vi "OFET2.vi"() -> ()   [LabVIEW 2017]
uses:
  EnumEstados1.ctl
  <vilib>/Analysis/3filter.llb/Filter Passband Type.ctl
  <vilib>/Analysis/baseanly.llb/IIR Cascade Filter (DBL).vi
  <vilib>/Analysis/NI_AALBase.lvlib
  <vilib>/Utility/NIReport.llb/NI_report.lvclass
  <vilib>/addons/_office/NI_ReportGenerationToolkit.lvlib
  <vilib>/addons/_office/excel.llb/Excel Easy Table (str).vi
panel:
  in  "Tab Control":T1(tab)
  in  "Voltaje final:  2":dbl=5.0
  in  "Voltaje inicial:  2":dbl
  in  "Paso: 2":dbl
  in  "Voltaje final:":dbl=5.0
  in  "Voltaje inicial:":dbl
  in  "Paso:":dbl=0.1
  in  "Paso":dbl
  in  "Voltaje inicial:":dbl
  in  "Voltaje final:":dbl
  in  "Voltaje:":dbl
  in  "order":i32
  in  "Stop Button":bool
  in  "Save Button":bool
  in  "Guardar en:":path
  out "Voltage-Current Characterization:":cluster{dbl[], "Filtered X":dbl[]}(graph)
  in  "Ok":bool
  # "OFET"
  # "VGS"
  # "VDS"
  # "VGS"
  # "VDS"
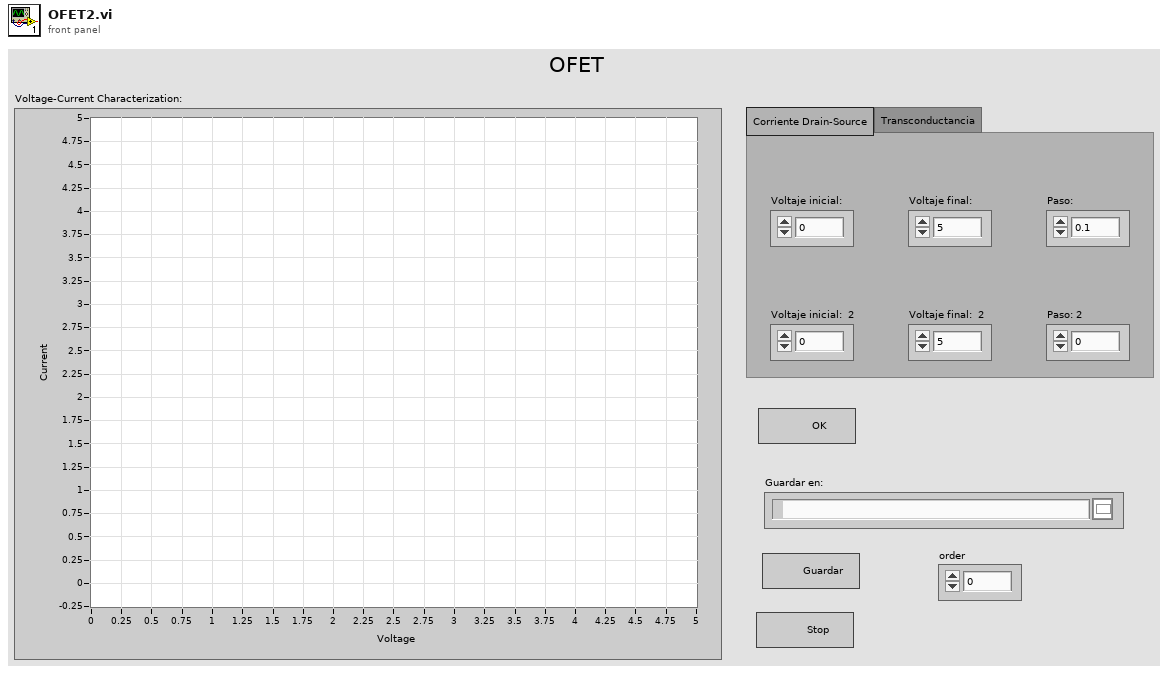
[diagram p1: front panel]
types:
  T1 = enum32{"Corriente Drain-Source", "Transconductancia"}
  T2 = typedef "EnumEstados1.ctl" = enum16{"Inicio", "LecturaDatos", "Cierre"}
  T3 = typedef "NI_AALBase.lvlib/Filter Passband Type.ctl" = enum32{"Lowpass", "Highpass", "Bandpass", "Bandstop"}
  T4 = enum16{"Standard Report", "HTML", "Word", "Excel"}
  T5 = enum16{"maximized", "minimized", "normal", "no change"}
  T6 = enum16{"open", "open or create", "create or replace", "create", "open (read-only)"}
  T7 = cluster{"task out":refnum<k21>, "error out":errorcluster}
  T8 = cluster{"filter structure":enum32{"IIR 2nd Order", "IIR 4th Order"}, "Reverse Coefficients":dbl[], "Forward Coefficients":dbl[]}
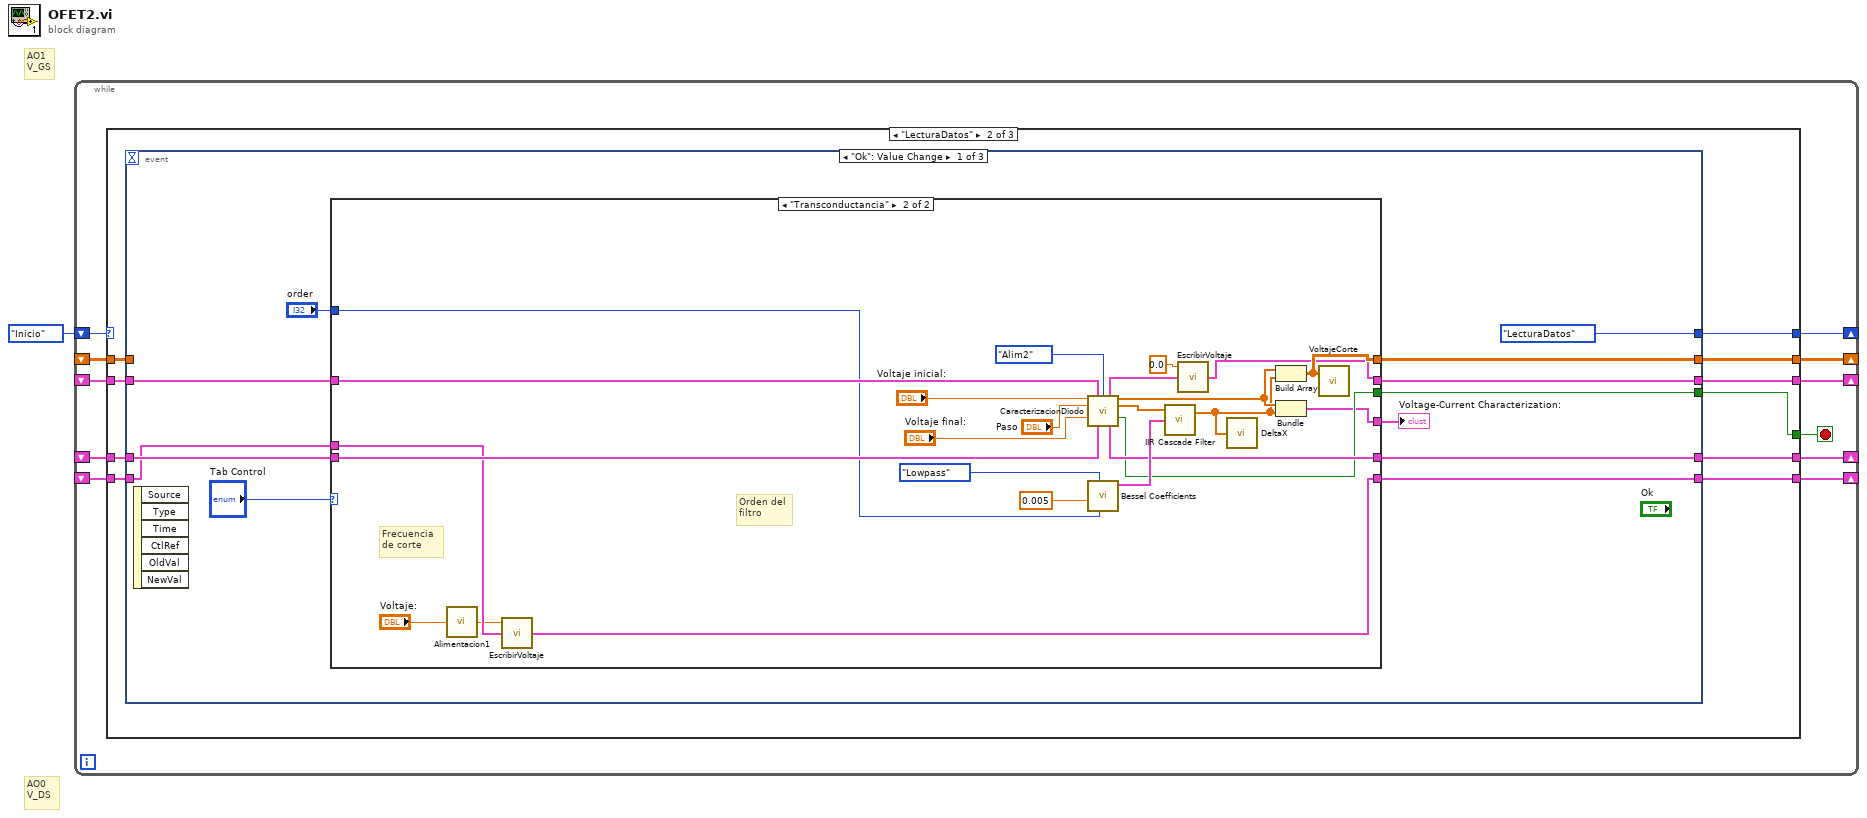
[diagram p0: block diagram]
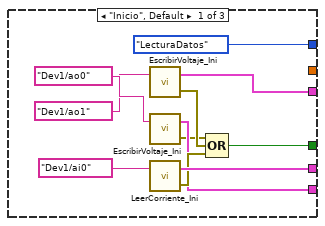
[diagram p2: hidden frame]
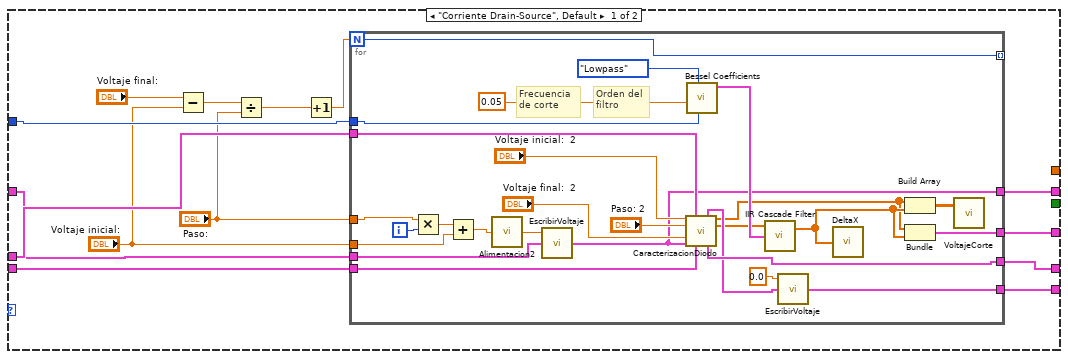
[diagram p3: hidden frame]
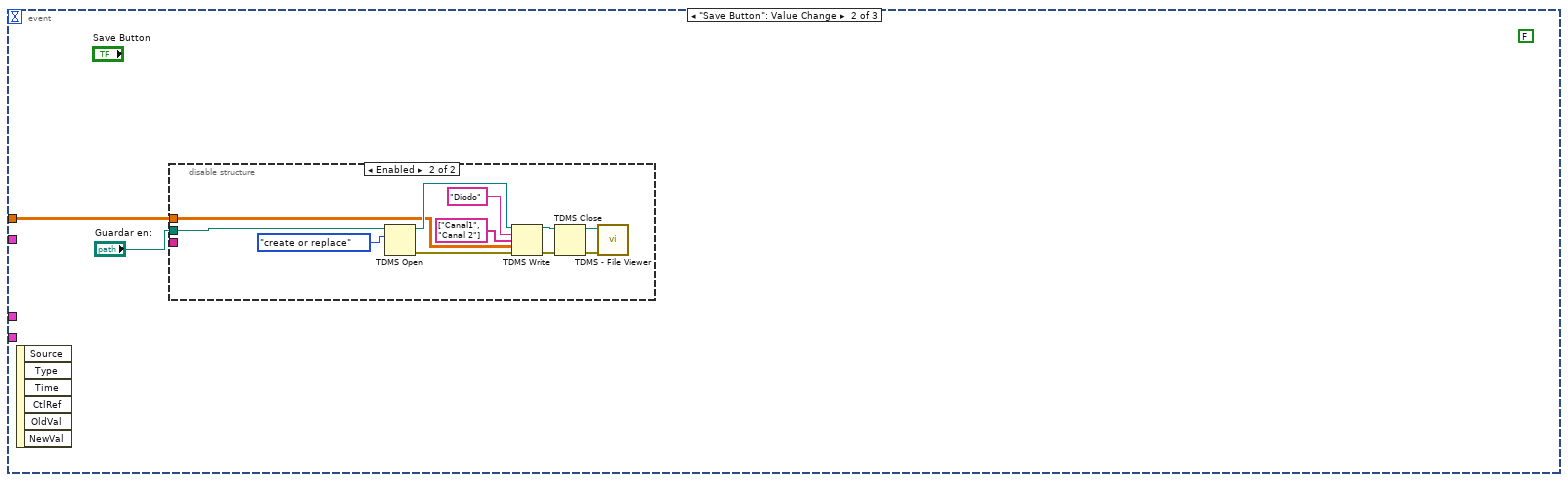
[diagram p4: hidden frame]
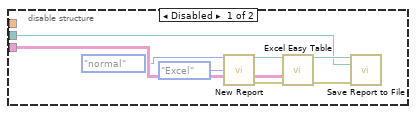
[diagram p5: hidden frame]
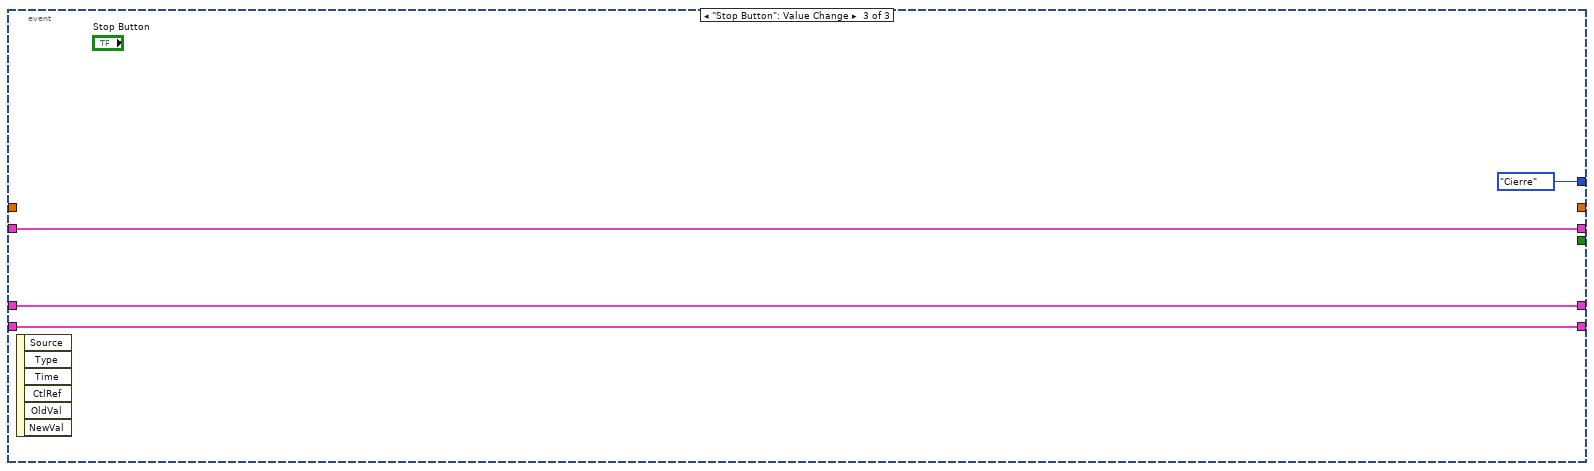
[diagram p6: hidden frame]
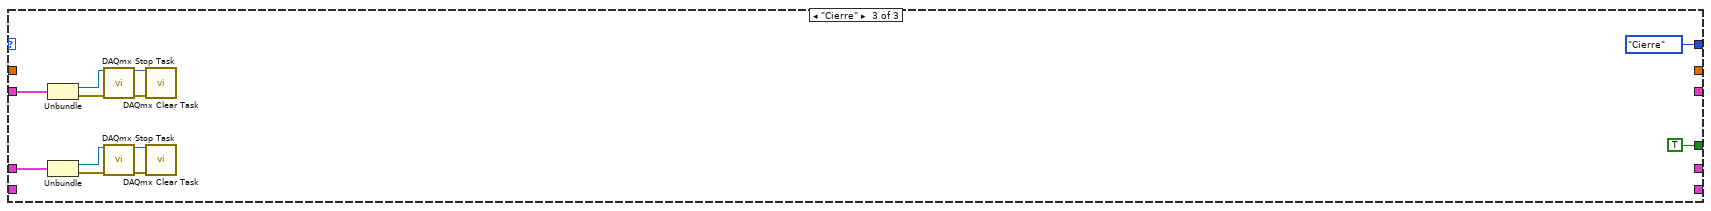
[diagram p7: hidden frame]
diagram:
  # "AO1\nV_GS"
  # "AO0\nV_DS"
  n1 = while {
    shift-right: [w7] -> _
    shift-left: EnumEstados1."Inicio" -> [w12]
    shift-right: [w11] -> _
    shift-left: _ -> [w10]
    shift-right: [w9] -> _
    shift-left: _ -> [w8]
    shift-right: [w6] -> _
    shift-left: _ -> [w5]
    shift-right: [w3] -> _
    shift-left: _ -> [w2]
    stop <- w4 stop-if-true
    n2 = case shown="\"LecturaDatos\"" w12 {
      tunnel: [w22 w32 _] -> w11
      tunnel: w10 -> [_ w33 w143]
      tunnel: [w21 w30 _] -> w9
      tunnel: w8 -> [_ w31 w142]
      tunnel: [EnumEstados1."LecturaDatos" w29 EnumEstados1."Cierre"] -> w7
      tunnel: [_ w28 _] -> w6
      tunnel: w5 -> [_ w27 _]
      tunnel: [w18 w26 TRUE] -> w4
      tunnel: [w17 w24 _] -> w3
      tunnel: w2 -> [_ w25 _]
      frame "Inicio", Default {
        n3 = call "EscribirVoltaje_Ini.vi"("physical channels"=tag "Dev1/ao1") -> ("error out"=w20:errorcluster, "cluster"=w22:T7)  [unwired: 1 in]
        n4 = call "EscribirVoltaje_Ini.vi"("physical channels"=tag "Dev1/ao0") -> ("error out"=w16:errorcluster, "cluster"=w17:T7)  [unwired: 1 in]
        n5 = call "LeerCorriente_Ini.vi"("physical channels"=tag "Dev1/ai0") -> ("error out"=w19:errorcluster, "output cluster"=w21:T7)  [unwired: 1 in]
        n6 = Compound Arithmetic op=OR(w16, w20, w19) -> (w18:bool)
      }
      frame "LecturaDatos" {
        n7 = event shown="[0] \"Ok\": Value Change" {
          selector: _ -> [_ _ _]
          dyn-events: _ -> [_ _ _]
          timeout: _ -> [_ _ _]
          tunnel: w33 -> [w44 _ w135]
          tunnel: [w37 _ w135] -> w32
          tunnel: w31 -> [w43 _ w134]
          tunnel: [w42 _ w134] -> w30
          tunnel: [EnumEstados1."LecturaDatos" _ EnumEstados1."Cierre"] -> w29
          tunnel: [w40 _ _] -> w28
          tunnel: w27 -> [_ w111 _]
          tunnel: [w41 _ _] -> w26
          tunnel: w25 -> [w39 _ w132]
          tunnel: [w38 _ w132] -> w24
          event "Ok": Value Change {
            n8 = event-data() -> ()  [unwired: 1 in, 6 out]
            n9 = case shown="\"Transconductancia\"" "Tab Control" {
              tunnel: w44 -> [w53 w108]
              tunnel: w43 -> [w57 w107]
              tunnel: [w56 w106] -> w42
              tunnel: [_ w105] -> w41
              tunnel: [_ w104] -> w40
              tunnel: w39 -> [w58 w100]
              tunnel: [w55 w99] -> w38
              tunnel: [w52 w97] -> w37
              tunnel: "order" -> [w59 w91]
              tunnel: [w54 w90] -> w34
              frame "Corriente Drain-Source", Default {
                n10 = Subtract(x="Voltaje final:", y="Voltaje inicial:") -> (x-y=w50:dbl)
                n11 = Divide(x=w50, y="Paso:") -> (x/y=w49:dbl)
                n12 = Increment(x=w49) -> (x+1=w46:dbl)
                n13 = for {
                  N: w46 -> [w66]
                  tunnel: w59 -> [w81]
                  tunnel: w58 -> [w77]
                  tunnel: w57 -> [w76]
                  tunnel: [w75] -> w56
                  tunnel: [w73] -> w55
                  tunnel: [w69] -> w54
                  tunnel: w53 -> [w68]
                  tunnel: [w67] -> w52
                  tunnel: [w66] -> _ mode=indexing
                  tunnel: "Paso:" -> [w65]
                  tunnel: "Voltaje inicial:" -> [w62]
                  i -> [w64]
                  # "Frecuencia \nde corte"
                  # "Orden del\nfiltro"
                  n14 = Multiply(x=w65, y=w64) -> (x*y=w63:dbl)
                  n15 = Add(x=w63, y=w62) -> (x+y=w61:dbl)
                  n16 = call "Alimentacion2.vi"("VoltajeDeseado"=w61) -> ("Numeric Indicator"=w60:dbl)
                  n17 = call "EscribirVoltaje.vi"("cluster"=w68, "data"=w60) -> ("Cluster"=w67:T7)  [unwired: 1 in, 2 out]
                  n18 = call "CaracterizacionDiodo.vi"("Voltaje inicial:"="Voltaje inicial:  2", "Voltaje"=w77, "Paso"="Paso: 2", "Voltaje final:"="Voltaje final:  2", "Voltaje  2"=w67, "Corriente"=w76) -> (3:"Voltaje"=w74:T7, 4:"Voltaje"=w70:dbl[], 6:"Corriente"=w71:dbl[], 14:"Corriente"=w75:T7)  [unwired: 5 in, 1 out]
                  n19 = call <vilib>:"Bessel Coefficients.vi"("order"=w81, "filter type"=Filter_Passband_Type."Lowpass", "low cutoff freq: fl"=0.05 ("Numeric Control")) -> ("IIR Filter Cluster"=w86:T8)  [unwired: 7 in, 1 out]
                  n20 = call-poly <vilib>:"IIR Cascade Filter.vi"("IIR Filter Cluster"=w86, "X"=w71) -> ("Filtered X"=w83:dbl[])  [unwired: 1 in, 1 out]
                  n21 = call "EscribirVoltaje.vi"("cluster"=w74, "data"=0.0) -> ("Cluster"=w73:T7)  [unwired: 1 in, 2 out]
                  n22 = call "DeltaX.vi"("Array in"=w83) -> ()  [unwired: 1 out]
                  n23 = Build Array(w70, w83) -> (w84:dbl[][])
                  n24 = Bundle("Voltaje"=w70, "Filtered X"=w83) -> (w69:cluster{"Voltaje":dbl[], "Filtered X":dbl[]})  [unwired: 1 in]
                  n25 = call "VoltajeCorte.vi"("Array in"=w84) -> ()  [unwired: 1 in, 2 out]
                }
              }
              frame "Transconductancia" {
                # "Frecuencia \nde corte"
                # "Orden del\nfiltro"
                n26 = call "Alimentacion1.vi"("VoltajeDeseado"="Voltaje:") -> ("Numeric Indicator"=w88:dbl)
                n27 = call "EscribirVoltaje.vi"("cluster"=w100, "data"=w88) -> ("Cluster"=w99:T7)  [unwired: 1 in, 2 out]
                n28 = call "CaracterizacionDiodo.vi"("Voltaje inicial:"="Voltaje inicial:", "Voltaje"=w108, "Enum"=enum16{"Alim1", "Alim2"}."Alim2", "Paso"="Paso", "Voltaje final:"="Voltaje final:", "Corriente"=w107) -> (3:"Voltaje"=w98:T7, 4:"Voltaje"=w103:dbl[], 6:"Corriente"=w95:dbl[], "Error?"=w105:bool, 14:"Corriente"=w106:T7)  [unwired: 5 in]
                n29 = call <vilib>:"Bessel Coefficients.vi"("order"=w91, "filter type"=Filter_Passband_Type."Lowpass", "low cutoff freq: fl"=0.005 ("Numeric Control")) -> ("IIR Filter Cluster"=w110:T8)  [unwired: 7 in, 1 out]
                n30 = call-poly <vilib>:"IIR Cascade Filter.vi"("IIR Filter Cluster"=w110, "X"=w95) -> ("Filtered X"=w102:dbl[])  [unwired: 1 in, 1 out]
                n31 = call "EscribirVoltaje.vi"("cluster"=w98, "data"=0.0) -> ("Cluster"=w97:T7)  [unwired: 1 in, 2 out]
                n32 = call "DeltaX.vi"("Array in"=w102) -> ()  [unwired: 1 out]
                n33 = Build Array(w103, w102) -> (w104:dbl[][])
                n34 = Bundle("Voltaje"=w103, "Filtered X"=w102) -> (w90:cluster{"Voltaje":dbl[], "Filtered X":dbl[]})  [unwired: 1 in]
                n35 = call "VoltajeCorte.vi"("Array in"=w104) -> ()  [unwired: 1 in, 2 out]
              }
            }
            "Voltage-Current Characterization:" <- w34
          }
          event "Save Button": Value Change {
            (unwired) FALSE
            n36 = event-data() -> ()  [unwired: 1 in, 6 out]
            n37 = disable-structure shown="Enabled" {
              disable-tunnel: _ -> [w118 _]
              disable-tunnel: "Guardar en:" -> [w113 w124]
              disable-tunnel: w111 -> [_ w121]
              frame Disabled {
                n38 = call <vilib>:"New Report.vi"("window state (normal)"=T5."normal", "report type"=T4."Excel") -> ("report out"=w120:refnum<class "NI_report.lvclass">, "error out"=w119:errorcluster)  [unwired: 12 in]
                n39 = call-poly <vilib>:"Excel Easy Table.vi"("report in"=w120, "text data"=w118, "error in (no error)"=w119) -> ("report out"=w117:refnum<class "NI_report.lvclass">, "error out"=w116:errorcluster)  [unwired: 8 in, 3 out]
                n40 = call-dynamic "Save Report to File.vi"("report in"=w117, "report file path"=w113, "error in (no error)"=w116) -> ()  [unwired: 11 in, 2 out]
              }
              frame Enabled {
                n41 = TDMS Open(10:T6."create or replace" ("operation (0:open)"), 11:w124) -> (0:w128:errorcluster, 3:w125:refnum<k34>)  [unwired: 5 in]
                n42 = TDMS Write(0:w125, 5:"Diodo" ("group name in (Untitled)"), 7:string[] ["Canal1", "Canal 2"] ("channel name(s) in (Untitled)"), 9:w121, 11:w128) -> (4:w126:refnum<k34>, 15:w127:errorcluster)  [unwired: 1 in, 2 out]
                n43 = TDMS Close(8:w127, 11:w126) -> (0:w123:errorcluster, 3:w122:path)
                n44 = call <vilib>:"TDMS - File Viewer.vi"("error in (no error)"=w123, "file path"=w122) -> ()  [unwired: 4 in, 2 out]
              }
            }
          }
          event "Stop Button": Value Change {
            n45 = event-data() -> ()  [unwired: 1 in, 6 out]
          }
        }
      }
      frame "Cierre" {
        n46 = Unbundle(w143) -> ("task out"=w141:refnum<k21>, "error out"=w140:errorcluster)
        n47 = Unbundle(w142) -> ("task out"=w139:refnum<k21>, "error out"=w138:errorcluster)
        n48 = call <vilib>:"DAQmx Stop Task.vi"("task/channels in"=w141, "error in"=w140) -> ("task out"=w147:refnum<k21>, "error out"=w146:errorcluster)  [unwired: 12 in]
        n49 = call <vilib>:"DAQmx Stop Task.vi"("task/channels in"=w139, "error in"=w138) -> ("task out"=w145:refnum<k21>, "error out"=w144:errorcluster)  [unwired: 12 in]
        n50 = call <vilib>:"DAQmx Clear Task.vi"("task in"=w147, "error in"=w146) -> ()  [unwired: 13 in, 1 out]
        n51 = call <vilib>:"DAQmx Clear Task.vi"("task in"=w145, "error in"=w144) -> ()  [unwired: 13 in, 1 out]
      }
    }
  }
